vi "saveExperimentControlArray_v05.vi"(6 "saveFileName":string, 7 "filepath":path, 8 "error in":errorcluster, 9 "subVI":path, 10 "mainVI":path, 11 "control array in":refnum<vi>[](array[refnum])) -> (0 "error out":errorcluster, 3 "control array out":refnum<vi>[](array[refnum]))   [LabVIEW 2019]
panel:
  out "status":string
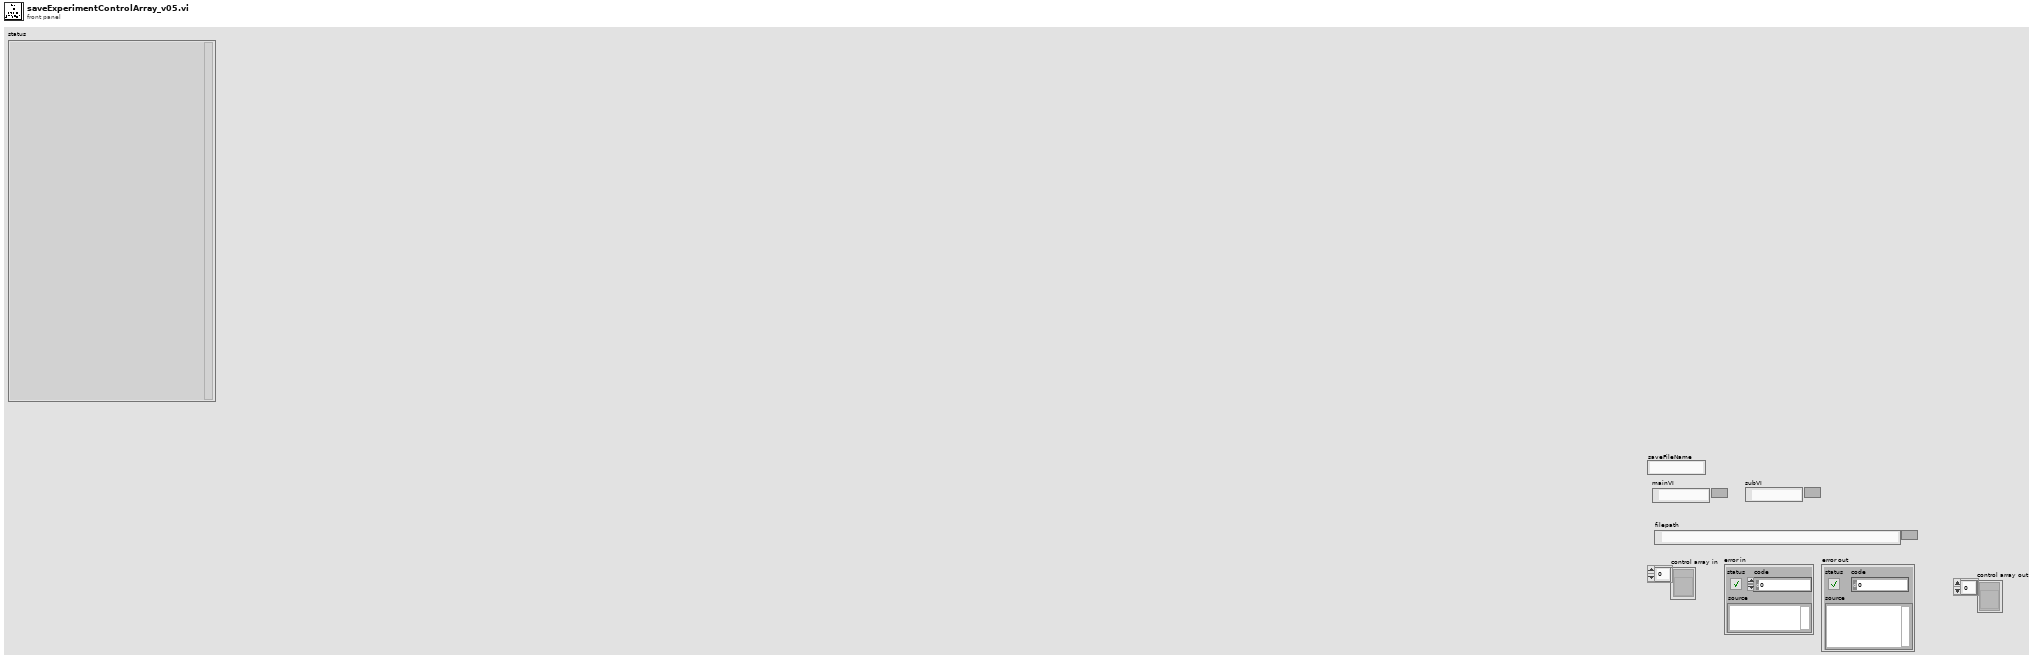
[diagram p1: front panel]
types:
  T1 = enum16{"open", "replace", "create", "open or create", "replace or create", "replace or create with confirmation"}
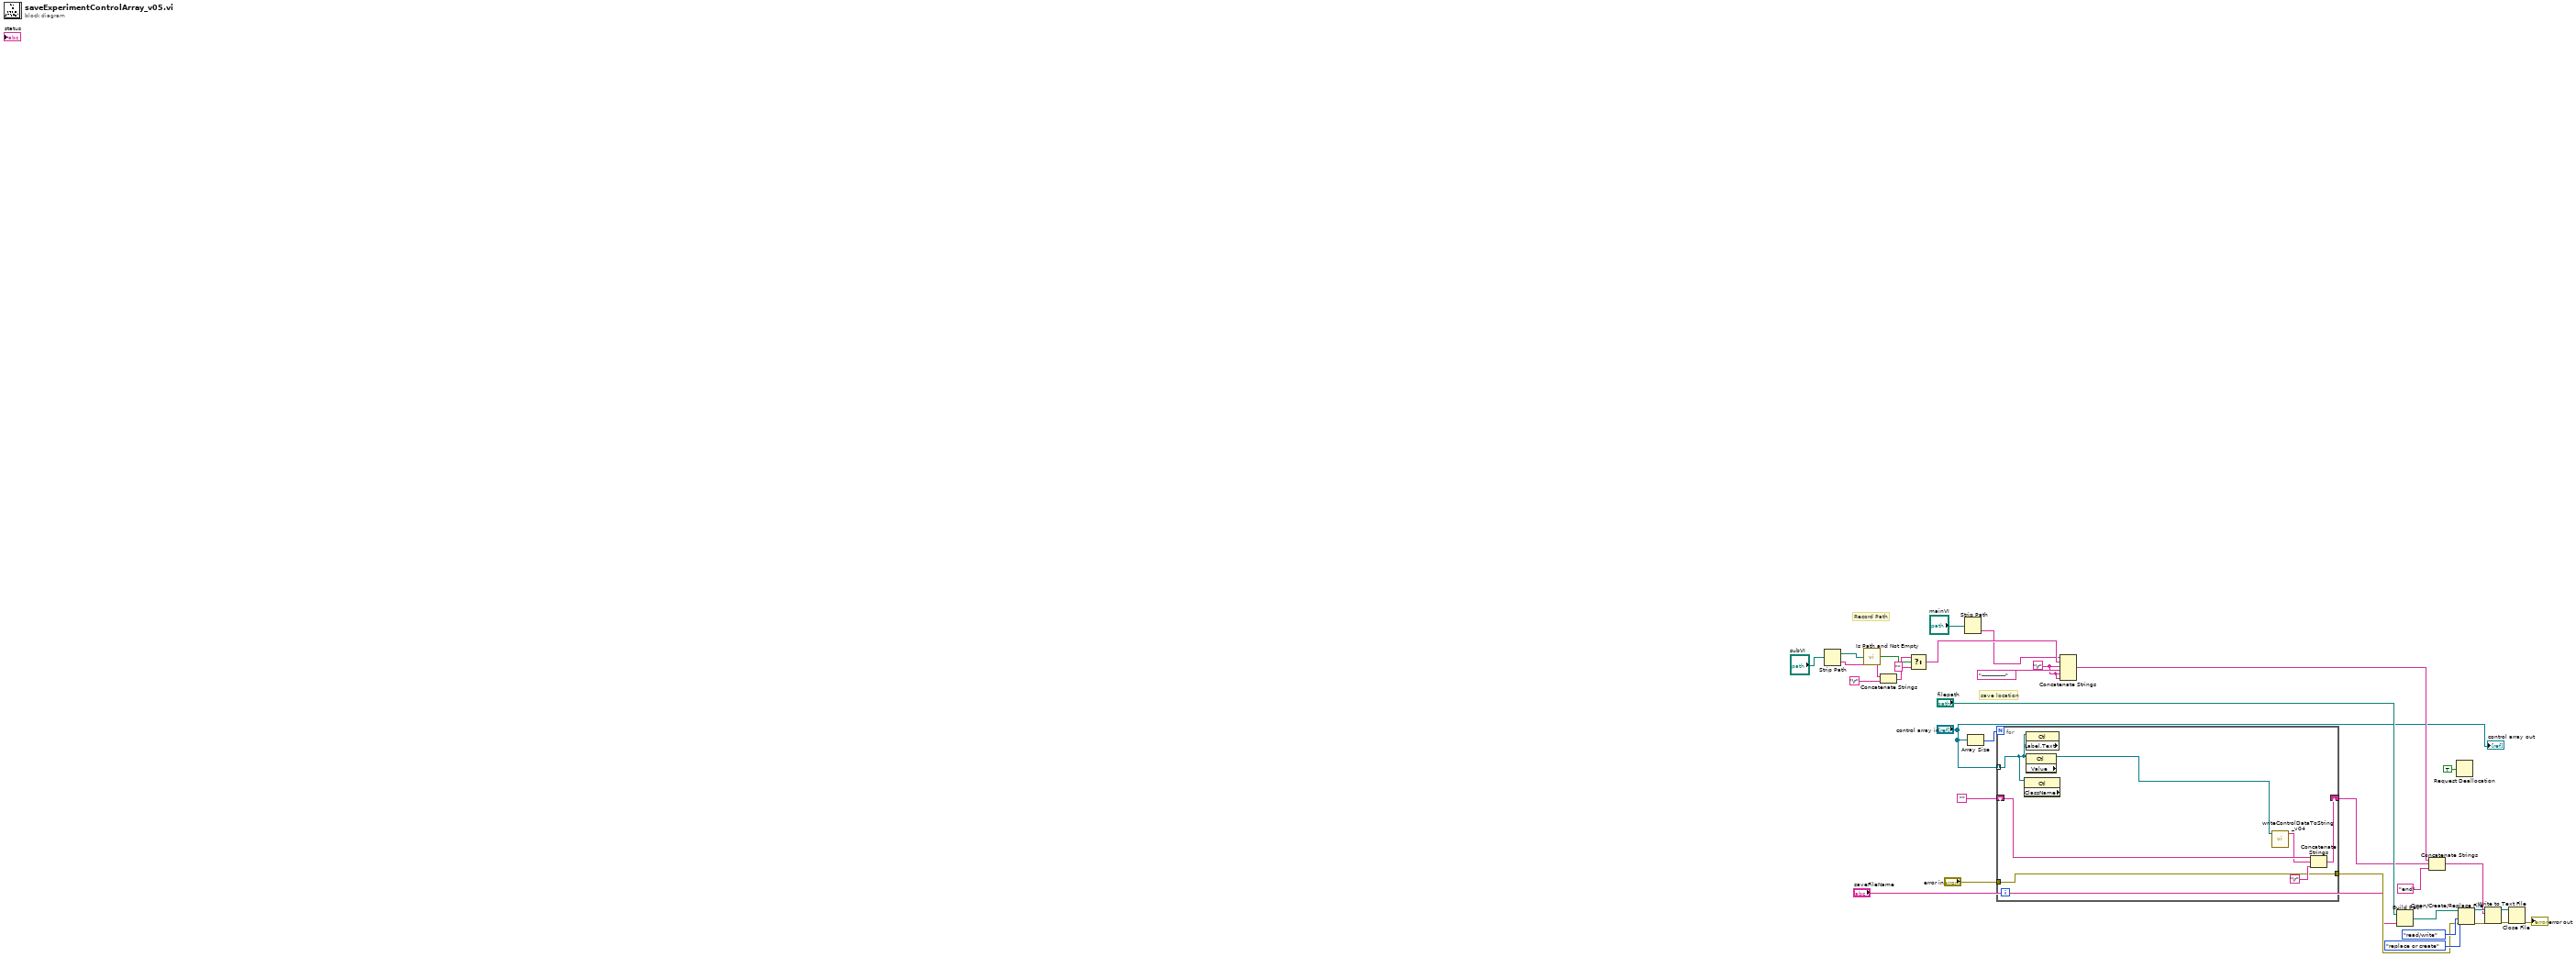
[diagram p0: block diagram]
diagram:
  w15 = "\r" ("string")
  # "save location"
  # "Record Path"
  n1 = Strip Path(path="subVI") -> (stripped path=w7:path, name=w6:string)
  n2 = call <vilib>:"Is Path and Not Empty.vi"("path"=w7) -> ("Is Path and Not Empty?"=w11:bool)  [unwired: 4 in]
  n3 = Concatenate Strings(w6, "\r" ("string")) -> (w12:string)
  n4 = Select(t=w12, s=w11, f="") -> (s? t:f=w9:string)
  n5 = Strip Path(path="mainVI") -> (name=w4:string)  [unwired: 1 out]
  n6 = Array Size(array="control array in") -> (size(s)=w23:i32)
  n7 = for {
    N: w23 -> [_]
    tunnel: "control array in" -> [w34] mode=indexing
    shift-right: [w38] -> w21
    shift-left: "" -> [w39]
    tunnel: "error in" -> [w36]
    tunnel: [w36] -> w17
    n8 = property class="Ctl" props=["ClassName"](reference=w34) -> ()  [unwired: 1 in, 3 out]
    n9 = property class="Ctl" props=["Label", "Text"](reference=w34) -> ()  [unwired: 1 in, 3 out]
    n10 = property class="Ctl" props=["Value"](reference=w34) -> (reference out=w35:refnum<vi>)  [unwired: 1 in, 2 out]
    n11 = call "writeControlDataToString_v04.vi"("Ctl Refnum"=w35) -> ("String written to file"=w33:string)  [unwired: 10 in]
    n12 = Concatenate Strings(w39, w33, "\r" ("string")) -> (w38:string)
  }
  n13 = Concatenate Strings(w4, w9, w15, "-------------" ("string"), w15, w15) -> (w14:string)
  n14 = Build Path(base path="filepath", name or relative path="saveFileName") -> (appended path=w32:path)
  n15 = Concatenate Strings(w14, w21, "end" ("string")) -> (w19:string)
  n16 = Request Deallocation(TRUE ("flag")) -> ()
  n17 = Open/Create/Replace File(file path (use dialog)=w32, error in=w17, operation (0:open)=T1."replace or create", access (0:read/write)=enum16{"read/write", "read-only", "write-only"}."read/write") -> (refnum out=w29:refnum<file>, error out=w30:errorcluster)  [unwired: 2 in, 1 out]
  n18 = Write to Text File(file (use dialog)=w29, text=w19, error in=w30) -> (refnum out=w27:refnum<file>, error out=w28:errorcluster)  [unwired: 1 in, 1 out]
  n19 = Close File(refnum=w27, error in=w28) -> (error out=→"error out":errorcluster)  [unwired: 1 out]
  "control array out" <- "control array in"
